vi "Part 2.vi"(11 "Input":string) -> (3 "Output":i64)   [LabVIEW 2021]
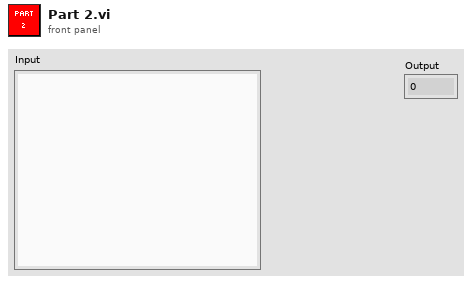
[diagram p1: front panel]
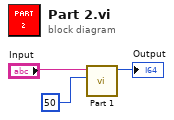
[diagram p0: block diagram]
diagram:
  n1 = call "Part 1.vi"("Iterations"=50, "Input"="Input") -> ("Output"=→"Output":i64)  [unwired: 9 in]
